vi "SendScriptToQueue.vi"(7 "Port":string, 9 "String":string, 11 "Queue in":refnum<queue>) -> ()   [LabVIEW 2016]
panel:
  # "The way it works - \n\nScript--- x\nx\nx\nx\nx\n\nCMD---\nCMD---"
  # "need the --- to execute it as a command and not send to REPL"
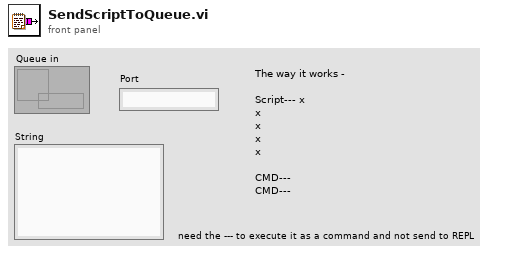
[diagram p1: front panel]
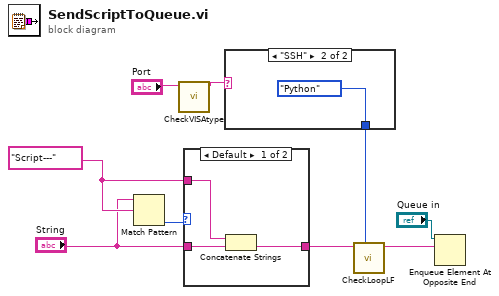
[diagram p0: block diagram]
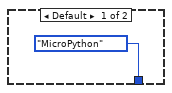
[diagram p2: hidden frame]
diagram:
  w7 = "Script---" ("write buffer")
  n1 = Match Pattern(string="String", regular expression=w7) -> (offset past match=w8:i32)  [unwired: 1 in, 3 out]
  n2 = call "CheckVISAtype.vi"("VISA Refnum in"="Port") -> ("data string"=w3:string)  [unwired: 8 in, 2 out]
  n3 = case shown="Default" w8 {
    tunnel: [w10 w13] -> w5
    tunnel: "String" -> [w11 w13]
    tunnel: w7 -> [w12 _]
    frame Default {
      n4 = Concatenate Strings(w12, w11) -> (w10:string)
    }
    frame 0..10 {
    }
  }
  n5 = case shown="\"SSH\"" w3 {
    tunnel: [enum16{"Python", "MicroPython"}."MicroPython" ("Code") enum16{"Python", "MicroPython"}."Python" ("Code")] -> w2
    frame Default {
    }
    frame "SSH" {
    }
  }
  n6 = call "CheckLoopLF.vi"(7:"Code"=w2, 11:"Code"=w5) -> ("Code fixed"=w4:string)  [unwired: 9 in]
  n7 = Enqueue Element At Opposite End(queue="Queue in", element=w4) -> ()  [unwired: 2 in, 3 out]
